vi "CanCoder_Execute.vi"   [LabVIEW 2023]
uses:
  <vilib>/Rock Robotics/WPI/ThirdParty/JAS_Junk/TrajLib/Util_GetTime.vi
  <vilib>/Rock Robotics/WPI/ThirdParty/JAS_Junk/TrajLib/VI/Util_GetTime_U32.vi
  <vilib>/Rock Robotics/SystemInterfaces/Utilities/FPGA_UtilitiesRead LocalTime.vi
  <vilib>/Rock Robotics/WPI/ThirdParty/JAS_Junk/TrajLib/VI/Util_GetTime_U64.vi
  <vilib>/Rock Robotics/Network Tables/NT Write Number.vi
  <vilib>/Rock Robotics/WPI/ThirdParty/JAS_Junk/TrajLib/Trajectory_Library.lvlib
  <vilib>/Rock Robotics/WPI/ThirdParty/Phoenix-LabVIEW/CANCoder/Get/CTRE_Phoenix_CANcoder_GetSensorData.vi
types:
  T1 = typedef "CTRE_Phoenix_CANcoder_DeviceRef.ctl" = cluster{"DeviceStatus":errorcluster, "Device Number":u8, "Handle":u64, "UsageFrame":u32, "Library Path":path}
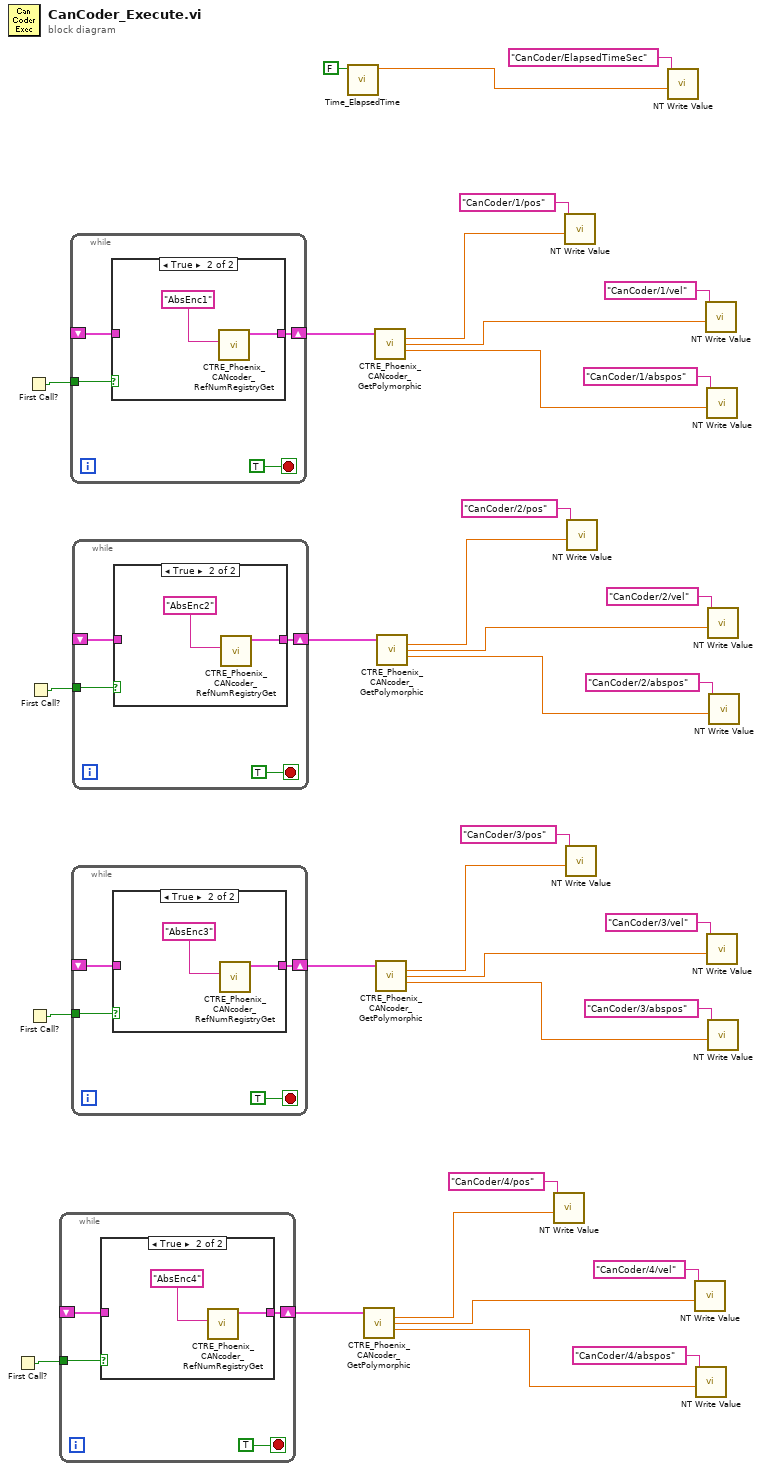
[diagram p0: block diagram]
diagram:
  n1 = First Call?() -> (First Call?: T/F=w8:bool)
  n2 = First Call?() -> (First Call?: T/F=w35:bool)
  n3 = First Call?() -> (First Call?: T/F=w16:bool)
  n4 = First Call?() -> (First Call?: T/F=w24:bool)
  n5 = while {
    tunnel: w8 -> [w37]
    shift-right: [w39] -> w4
    shift-left: _ -> [w36]
    stop <- TRUE stop-if-true
    n6 = case shown="True" w37 {
      tunnel: [w40 w42] -> w39
      tunnel: w36 -> [w40 _]
      frame False {
      }
      frame True {
        n7 = call <vilib>:"CTRE_Phoenix_CANcoder_RefNumRegistryGet.vi"("refnum name"="AbsEnc4") -> ("CTRE_CANcoder_DeviceRef"=w42:T1)  [unwired: 9 in, 1 out]
      }
    }
  }
  n8 = while {
    tunnel: w35 -> [w44]
    shift-right: [w46] -> w28
    shift-left: _ -> [w43]
    stop <- TRUE stop-if-true
    n9 = case shown="True" w44 {
      tunnel: [w47 w49] -> w46
      tunnel: w43 -> [w47 _]
      frame False {
      }
      frame True {
        n10 = call <vilib>:"CTRE_Phoenix_CANcoder_RefNumRegistryGet.vi"("refnum name"="AbsEnc1") -> ("CTRE_CANcoder_DeviceRef"=w49:T1)  [unwired: 9 in, 1 out]
      }
    }
  }
  n11 = while {
    tunnel: w16 -> [w51]
    shift-right: [w53] -> w12
    shift-left: _ -> [w50]
    stop <- TRUE stop-if-true
    n12 = case shown="True" w51 {
      tunnel: [w54 w56] -> w53
      tunnel: w50 -> [w54 _]
      frame False {
      }
      frame True {
        n13 = call <vilib>:"CTRE_Phoenix_CANcoder_RefNumRegistryGet.vi"("refnum name"="AbsEnc3") -> ("CTRE_CANcoder_DeviceRef"=w56:T1)  [unwired: 9 in, 1 out]
      }
    }
  }
  n14 = while {
    tunnel: w24 -> [w58]
    shift-right: [w60] -> w20
    shift-left: _ -> [w57]
    stop <- TRUE stop-if-true
    n15 = case shown="True" w58 {
      tunnel: [w61 w63] -> w60
      tunnel: w57 -> [w61 _]
      frame False {
      }
      frame True {
        n16 = call <vilib>:"CTRE_Phoenix_CANcoder_RefNumRegistryGet.vi"("refnum name"="AbsEnc2") -> ("CTRE_CANcoder_DeviceRef"=w63:T1)  [unwired: 9 in, 1 out]
      }
    }
  }
  n17 = call <vilib>:"Time_ElapsedTime.vi"("Reset"=FALSE) -> ("Elapsed Time Sec"=w30:dbl)  [unwired: 10 in]
  n18 = call-poly <vilib>:"CTRE_Phoenix_CANcoder_GetPolymorphic.vi"("CTRE_CANcoder_DeviceRef"=w4) -> ("Position"=w3:dbl, "Velocity"=w2:dbl, "Absolute Position"=w1:dbl)  [unwired: 10 in, 2 out]
  n19 = call-poly <vilib>:"CTRE_Phoenix_CANcoder_GetPolymorphic.vi"("CTRE_CANcoder_DeviceRef"=w28) -> ("Position"=w27:dbl, "Velocity"=w26:dbl, "Absolute Position"=w25:dbl)  [unwired: 10 in, 2 out]
  n20 = call-poly <vilib>:"CTRE_Phoenix_CANcoder_GetPolymorphic.vi"("CTRE_CANcoder_DeviceRef"=w12) -> ("Position"=w11:dbl, "Velocity"=w10:dbl, "Absolute Position"=w9:dbl)  [unwired: 10 in, 2 out]
  n21 = call-poly <vilib>:"CTRE_Phoenix_CANcoder_GetPolymorphic.vi"("CTRE_CANcoder_DeviceRef"=w20) -> ("Position"=w19:dbl, "Velocity"=w18:dbl, "Absolute Position"=w17:dbl)  [unwired: 10 in, 2 out]
  n22 = call-poly <vilib>:"NT Write Value.vi"("value"=w3, "name"="CanCoder/4/pos") -> ()  [unwired: 9 in, 1 out]
  n23 = call-poly <vilib>:"NT Write Value.vi"("value"=w27, "name"="CanCoder/1/pos") -> ()  [unwired: 9 in, 1 out]
  n24 = call-poly <vilib>:"NT Write Value.vi"("value"=w11, "name"="CanCoder/3/pos") -> ()  [unwired: 9 in, 1 out]
  n25 = call-poly <vilib>:"NT Write Value.vi"("value"=w19, "name"="CanCoder/2/pos") -> ()  [unwired: 9 in, 1 out]
  n26 = call-poly <vilib>:"NT Write Value.vi"("value"=w30, "name"="CanCoder/ElapsedTimeSec") -> ()  [unwired: 9 in, 1 out]
  n27 = call-poly <vilib>:"NT Write Value.vi"("value"=w2, "name"="CanCoder/4/vel") -> ()  [unwired: 9 in, 1 out]
  n28 = call-poly <vilib>:"NT Write Value.vi"("value"=w1, "name"="CanCoder/4/abspos") -> ()  [unwired: 9 in, 1 out]
  n29 = call-poly <vilib>:"NT Write Value.vi"("value"=w26, "name"="CanCoder/1/vel") -> ()  [unwired: 9 in, 1 out]
  n30 = call-poly <vilib>:"NT Write Value.vi"("value"=w25, "name"="CanCoder/1/abspos") -> ()  [unwired: 9 in, 1 out]
  n31 = call-poly <vilib>:"NT Write Value.vi"("value"=w10, "name"="CanCoder/3/vel") -> ()  [unwired: 9 in, 1 out]
  n32 = call-poly <vilib>:"NT Write Value.vi"("value"=w18, "name"="CanCoder/2/vel") -> ()  [unwired: 9 in, 1 out]
  n33 = call-poly <vilib>:"NT Write Value.vi"("value"=w9, "name"="CanCoder/3/abspos") -> ()  [unwired: 9 in, 1 out]
  n34 = call-poly <vilib>:"NT Write Value.vi"("value"=w17, "name"="CanCoder/2/abspos") -> ()  [unwired: 9 in, 1 out]
